vi "Create_Probe_Box.vi"(1 "Probe Volume":T1=[{"Max"=15.0, "Min"=-15.0}, {"Max"=250.0, "Min"=0.0}, {"Max"=15.0, "Min"=-15.0}] {"Min" format="%#.1f"; "Max" format="%#.1f"}, 2 "Probe Position":dbl[](array[numeric]) format="%.2f") -> (0 "Current Probe Volume":cluster{"Max":dbl, "Min":dbl}[](array[cluster])=[{"Max"=15015.0, "Min"=14985.0}, {"Max"=550.0, "Min"=300.0}, {"Max"=35.0, "Min"=5.0}] {"Min" format="%.2f"; "Max" format="%.2f"})   [LabVIEW 2010]
uses:
  Box_size.ctl
panel:
  # "(Relative to measurement position)"
  # "X                           Y                          Z"
  # "X                Y                  Z"
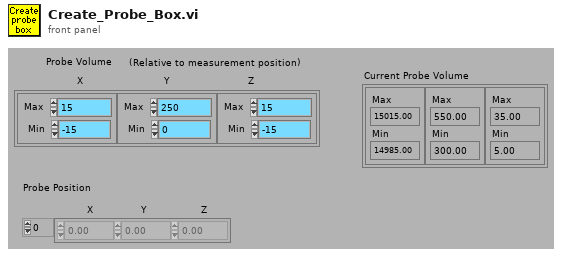
[diagram p1: front panel]
types:
  T1 = typedef "Box_size.ctl" = cluster{"Max":dbl, "Min":dbl}[]
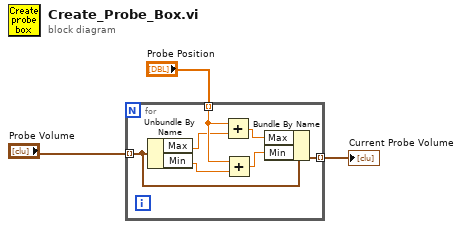
[diagram p0: block diagram]
diagram:
  n1 = for {
    tunnel: "Probe Volume" -> [w7] mode=indexing
    tunnel: "Probe Position" -> [w10] mode=indexing
    tunnel: [w4] -> w1 mode=indexing
    n2 = Unbundle By Name(w7) -> ("Max"=w9:dbl, "Min"=w8:dbl)
    n3 = Add(x=w10, y=w9) -> (x+y=w6:dbl)
    n4 = Add(x=w10, y=w8) -> (x+y=w5:dbl)
    n5 = Bundle By Name(cluster=w7, "Max"=w6, "Min"=w5) -> (w4:cluster{"Max":dbl, "Min":dbl})
  }
  "Current Probe Volume" <- w1
